vi "灰度直方图分析2.vi"() -> ()   [LabVIEW 2018]
uses:
  <vilib>/vision/NI_Vision_Development_Module.lvlib
panel:
  out "error out 2":errorcluster
  out "Histogram Report":T1 {"Standard  Variation" format="%.2f"; "Mean Value" format="%.2f"; "Interval Width" format="%.2f"; "Starting Value" format="%.2f"; "Maximal Value" format="%.2f"; "Minimal Value" format="%.2f"}
  out "灰度图":T2(graph)
  out "error out":errorcluster
  out "Standard  Deviation":sgl format="%.2f"
  out "Mean Value":sgl format="%.2f"
  out "Histogram Graph":T2 {"Incremental Value" format="%.2f"; "Starting Value" format="%.2f"}
  out "Image":T3(plugin-control)
  in  "路径":path
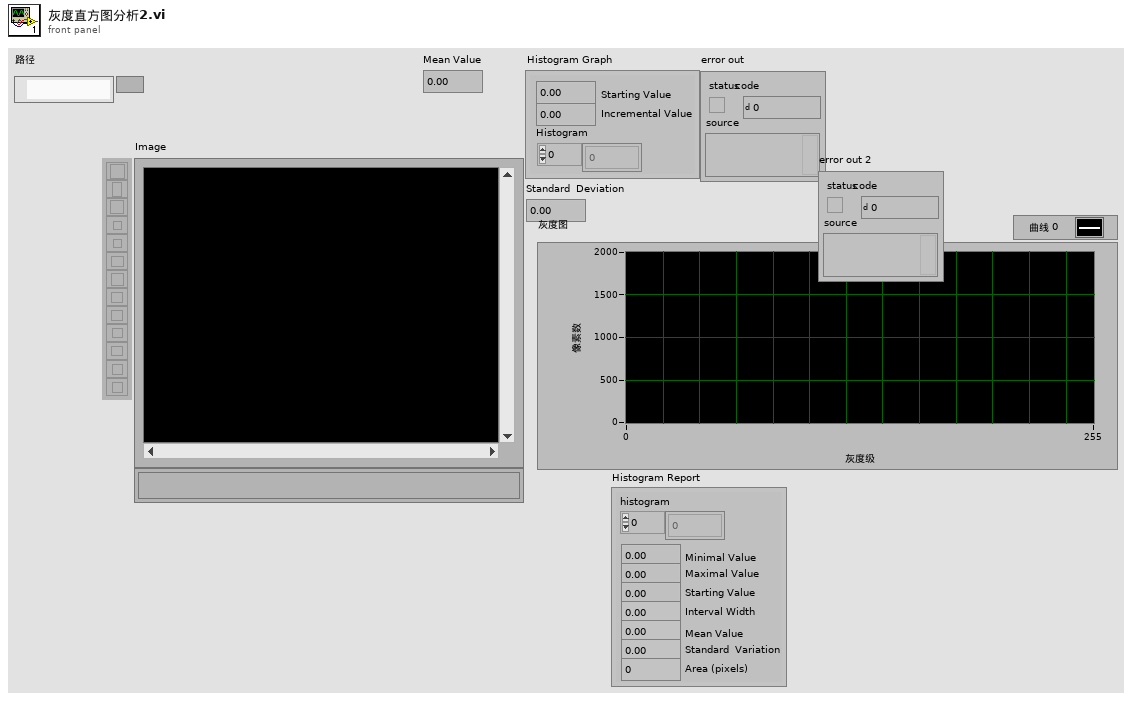
[diagram p1: front panel]
types:
  T1 = cluster{"histogram":u32[], "Minimal Value":sgl, "Maximal Value":sgl, "Starting Value":sgl, "Interval Width":sgl, "Mean Value":sgl, "Standard  Variation":sgl, "Area (pixels)":i32}
  T2 = cluster{"Starting Value":sgl, "Incremental Value":sgl, "Histogram":u32[]}
  T3 = typedef "IMAQ Image.ctl" = refnum<image>
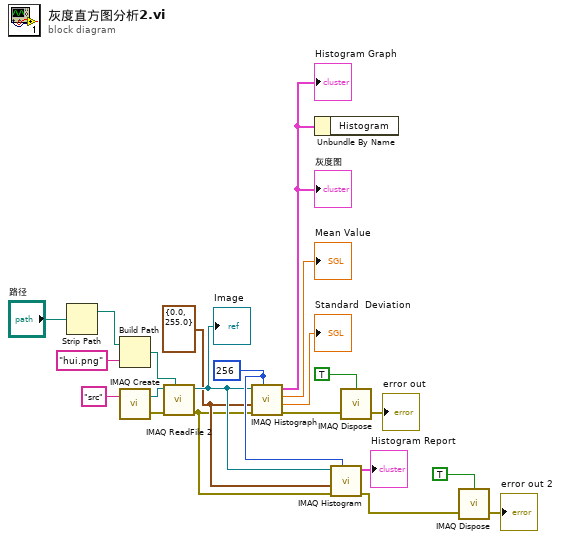
[diagram p0: block diagram]
diagram:
  w6 = cluster{"Minimum":sgl, "Maximum":sgl} {"Minimum"=0.0, "Maximum"=255.0} ("Interval Range")
  w8 = 256 ("Number of Classes")
  n1 = Strip Path(path="路径") -> (stripped path=w21:path)  [unwired: 1 out]
  n2 = Build Path(base path=w21, name or relative path="hui.png" ("名称或相对路径")) -> (appended path=w19:path)
  n3 = call "IMAQ Create"("Image Name"="src") -> ("New Image"=w17:T3, "error out"=w9:errorcluster)  [unwired: 4 in]
  n4 = call "IMAQ ReadFile 2"("File Path"=w19, "error in (no error)"=w9, "Image"=w17) -> ("error out"=w5:errorcluster, "Image Out"=w7:T3)  [unwired: 4 in, 3 out]
  "Image" <- w7
  n5 = call "IMAQ Histograph"("Number of Classes"=w8, "error in (no error)"=w5, "Interval Range"=w6, "Image"=w7) -> ("error out"=w13:errorcluster, "Standard  Deviation"=→"Standard  Deviation":sgl, "Mean Value"=→"Mean Value":sgl, "Histogram Graph"=w10:T2)  [unwired: 4 in]
  "Histogram Graph" <- w10
  "灰度图" <- w10
  n6 = Unbundle By Name(w10) -> ()  [unwired: 1 out]
  n7 = call "IMAQ Histogram"("Number of Classes"=w8, "error in (no error)"=w5, "Interval Range"=w6, "Image"=w7) -> ("error out"=w2:errorcluster, "Histogram Report"=→"Histogram Report":T1)  [unwired: 6 in]
  n8 = call "IMAQ Dispose"("All Images? (No)"=TRUE, "error in (no error)"=w13) -> ("error out"=→"error out":errorcluster)  [unwired: 4 in]
  n9 = call "IMAQ Dispose"("All Images? (No)"=TRUE, "error in (no error)"=w2) -> ("error out"=→"error out 2":errorcluster)  [unwired: 4 in]
